vi "ge_NumInputCols.vi"(0 "MeasType":T2, 1 "ge_DAQManDefinitions":T1) -> (6 "Max Input Col":i32)   [LabVIEW 2018]
uses:
  Custom Ctrls/ge_MeasType.ctl
  Common/Controls/DAQMan Definitions.ctl
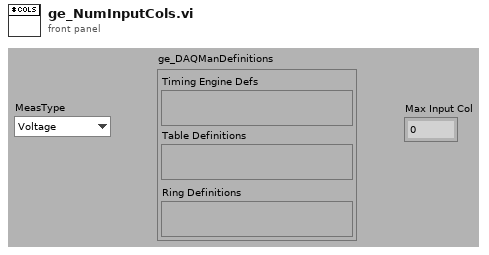
[diagram p1: front panel]
types:
  T1 = typedef "DAQMan Definitions.ctl" = cluster{"Timing Engine Defs":variant, "Table Definitions":variant, "Ring Definitions":variant}
  T2 = typedef "ge_MeasType.ctl" = enum16{"Voltage", "Frequency", "Tachometer", "Dynamic", "Thermocouple", "RTD", "Strain", "Current", "Resistance"}
  T3 = typedef "ge_ColDef.ctl" = cluster{"ge_HdrNames":T4, "HdrInfo":T5}
  T4 = typedef "HeaderNames.ctl" = enum16{"Channel", "Device", "Spacer", "Description", "MB", "Range", "Terminal", "Coupling", "Thresh (V)", "Pulse/Rev", "Slope", "Min EU", "Min RPM", "mV/EU", "Iex", "Temp Units", "Type", "CJC Src", "CJC Val", "Ro", "Wire Cfg", "Strain Mode", "Vex", "Bridge Type", "GF", "Gauge Res", "Poisson", "Lead Res", "Init Strain", "GAF", "Scale", "Offset", "Unit (EU)", "dB?", "dB Ref", "Cal Mag", "Cal Units", "Max Temp", "Min Temp", "Max Strain", "Min Strain"}
  T5 = typedef "ge_HdrInfo.ctl" = cluster{"Hdr Width":i32, "Glbl Ctrl":T6}
  T6 = typedef "ge_GlblCtrls.ctl" = enum16{"Str0", "Bool0", "Bool1", "Int0", "Ring0", "Ring1", "Ring2", "Ring3", "Dbl0", "Dbl1", "Dbl2", "Dbl3", "Cal0", "Cal1", "Cal2", "None"}
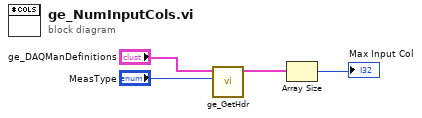
[diagram p0: block diagram]
diagram:
  n1 = call "ge_GetHdr.vi"("MeasType"="MeasType", "ge_DAQManDefinitions"="ge_DAQManDefinitions") -> ("Table Hdrs"=w2:T3[])  [unwired: 8 in, 1 out]
  n2 = Array Size(array=w2) -> (size(s)=→"Max Input Col":i32)
